vi "test performance.vi"(8 "error in (no error)":errorcluster) -> (0 "error out":errorcluster, 2 "ms Avg Dump":dbl, 3 "ms Avg Load":dbl)   [LabVIEW 2018, in "labview_json_tests.lvlib"]
uses:
  labview_json_tests.lvlib
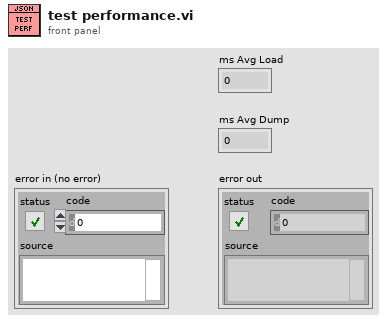
[diagram p1: front panel]
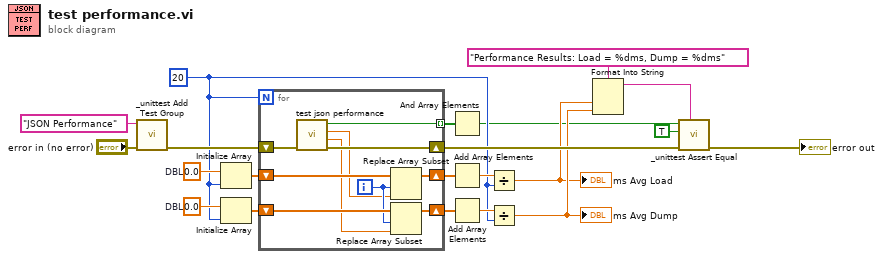
[diagram p0: block diagram]
diagram:
  w13 = 0.0  # DBL
  w14 = 0.0  # DBL
  w6 = 20
  n1 = call "_unittest Add Test Group.vi"("error in (no error)"="error in (no error)", "Test Group"="JSON Performance" ("Test Case")) -> ("error out"=w18:errorcluster)  [unwired: 9 in]
  n2 = Initialize Array(w14, w6) -> (w12:dbl[])
  n3 = Initialize Array(w13, w6) -> (w11:dbl[])
  n4 = for {
    N: w6 -> [_]
    shift-right: [w25] -> w17
    shift-left: w18 -> [w26]
    shift-right: [w29] -> w8
    shift-left: w11 -> [w30]
    shift-right: [w28] -> w10
    shift-left: w12 -> [w31]
    tunnel: [w24] -> w2 mode=indexing
    i -> [w27]
    n5 = call "test json performance.vi"("error in (no error)"=w26) -> ("error out"=w25:errorcluster, "ms Avg Dump"=w23:dbl, "ms Avg Load"=w22:dbl, "Passed?"=w24:bool)  [unwired: 7 in]
    n6 = Replace Array Subset(array=w31, new element=w22, index=w27) -> (w28:dbl[])
    n7 = Replace Array Subset(array=w30, new element=w23, index=w27) -> (w29:dbl[])
  }
  n8 = And Array Elements(Boolean array=w2) -> (logical AND=w1:bool)
  n9 = Add Array Elements(numeric array=w10) -> (sum=w9:dbl)
  n10 = Add Array Elements(numeric array=w8) -> (sum=w7:dbl)
  n11 = Divide(x=w9, y=w6) -> (x/y=w4:dbl)
  "ms Avg Load" <- w4
  n12 = Divide(x=w7, y=w6) -> (x/y=w5:dbl)
  "ms Avg Dump" <- w5
  n13 = Format Into String(format string="Performance Results: Load = %dms, Dump = %dms" ("Message"), w4, w5) -> (resulting string=w15:string)  [unwired: 2 in, 1 out]
  n14 = call "_unittest Assert Equal.vi"("Test Name"=w15, "error in (no error)"=w17, "Expected Value"=TRUE, "Actual Value"=w1) -> ("error out"=→"error out":errorcluster)  [unwired: 5 in, 2 out]
